vi "Parameters Import Action - Create Chans.v.vi"(8 "error in (no error)":errorcluster, 9 "Param ID map":map{i32, string}(c390), 10 "selected path":path, 11 "Item Ref in":T1 format="%.0x") -> (0 "error out":errorcluster, 2 "selected path out":path caption="selected path", 3 "Item Ref out":T1 format="%.0x")   [LabVIEW 2020, in "Ballard 1553 System Explorer.lvlib"]
uses:
  Ballard 1553 System Explorer.lvlib
  Shared/Controls and Global/Global.vi
  Shared/Ballard 1553 Shared.lvlib
  <vilib>/NI VeriStand/Custom Device Tools/Custom Device Utility Library/Custom Device Utility Library.lvlib
  <vilib>/NI VeriStand/Custom Device API/Custom Device API.lvlib
  c73aaead-b91a-4278-bfe3-fb22b68f848a.vi
  <vilib>/NI VeriStand/Custom Device Tools/Custom Device Utility Library/NI VeriStand - Search for All Items by GUID.vi
  1876eacf-d948-401b-a296-273bf559280d.vi
  <vilib>/NI VeriStand/Custom Device API/Custom Device Item Ref.ctl
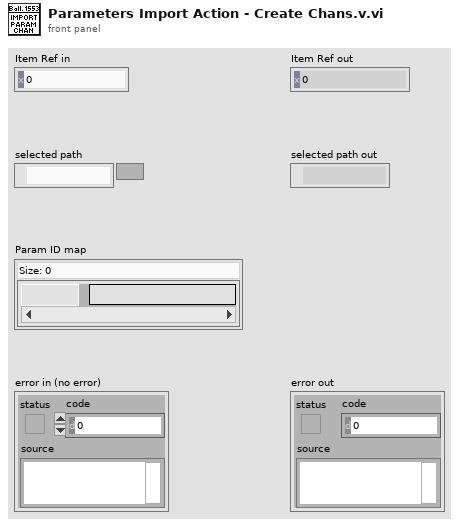
[diagram p1: front panel]
types:
  T1 = typedef "Custom Device API.lvlib/Custom Device Item Ref.ctl" = u64
  T2 = typedef "Ballard 1553 System Explorer.lvlib/param_sysdef_type.ctl" = cluster{"Num_Words":u8, "IDs":string[], "Parameter Map":map{string, cluster{"ICD_Signal_Name":string, "Type":enum16{"Opaque", "Enum", "Float", "Integer", "Bcd", "Bool"}, "Units":string, "Nword":i32, "StartBit":i32, "Size":i32, "LSB_Value":dbl, "Offset":i32, "Encoding":enum16{"None", "2-complement", "Unsigned"}}[]}}
  T3 = typedef "Custom Device API.lvlib/Custom Device Item Info.ctl" = cluster{"Name":string, "Is Channel":bool, "GUID":string, "Is Waveform":bool}
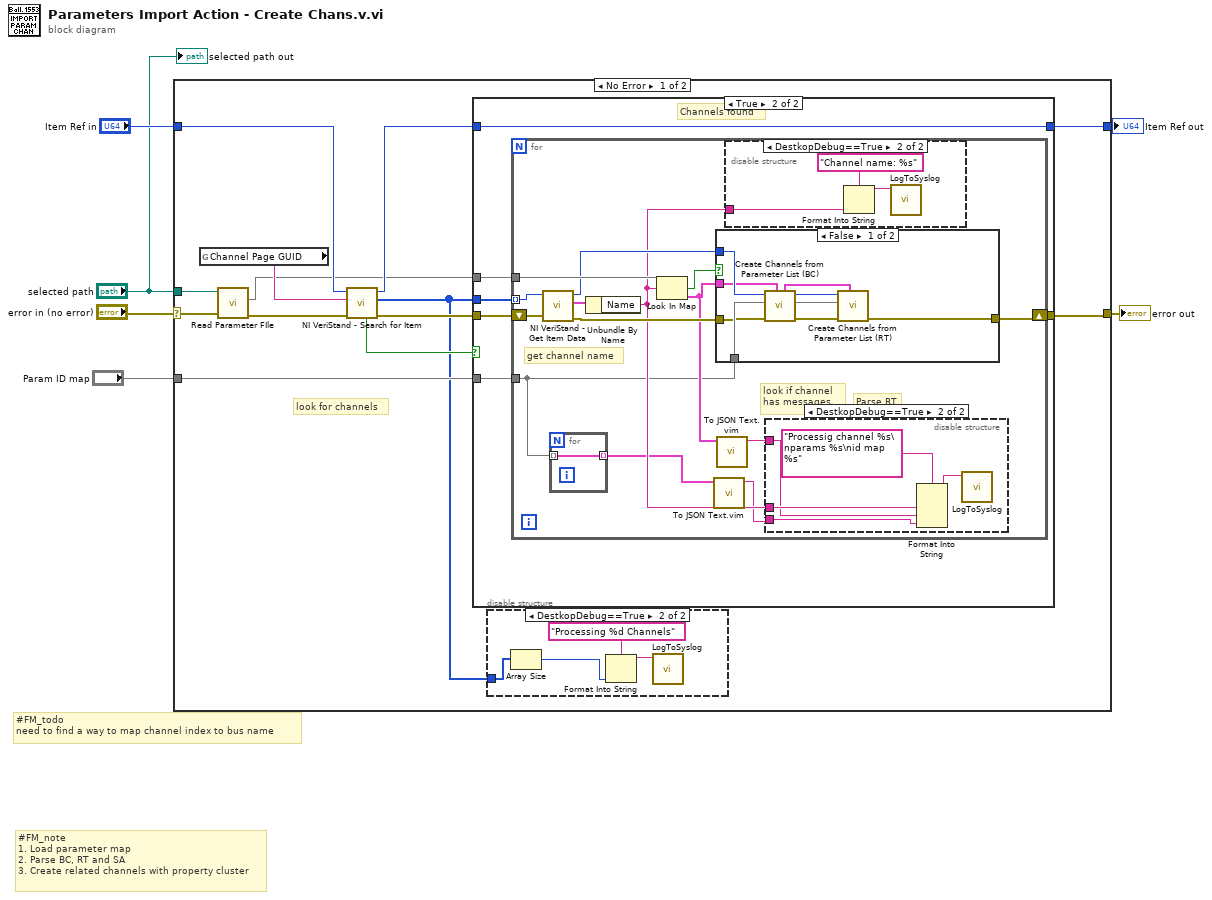
[diagram p0: block diagram]
diagram:
  # "#FM_todo\nneed to find a way to map channel index to bus name"
  # "#FM_note \n1. Load parameter map\n2. Parse BC, RT and SA\n3. Create related channels with property cluster"
  n1 = case shown="No Error" "error in (no error)" {
    selector: "error in (no error)" -> [w18 w65]
    tunnel: "selected path" -> [w19 _]
    tunnel: [w9 w66] -> w5
    tunnel: "Item Ref in" -> [w17 w66]
    tunnel: [w10 w65] -> w3
    tunnel: "Param ID map" -> [w11 _]
    frame No Error {
      # "look for channels"
      n2 = global read "Global.vi" "Channel Page GUID"() -> (w15:string)
      n3 = call "Read Parameter FIle.vi"("error in"=w18, "path in"=w19) -> ("error out"=w16:errorcluster, "Parameter map"=w8:map{string, T2})  [unwired: 7 in, 1 out]
      n4 = call-poly <vilib>:"NI VeriStand - Search for Item.vi"("error in"=w16, "Item GUID"=w15, "Section Ref in"=w17) -> ("error out"=w12:errorcluster, "Item Refs"=w7:T1[], "Section Ref out"=w14:T1, "Found"=w13:bool)  [unwired: 5 in]
      n5 = case shown="True" w13 {
        tunnel: w14 -> [w24 w27]
        tunnel: w7 -> [_ w30]
        tunnel: w12 -> [w25 w31]
        tunnel: w11 -> [_ w29]
        tunnel: [w25 w28] -> w10
        tunnel: [w24 w27] -> w9
        tunnel: w8 -> [_ w26]
        frame False {
        }
        frame True {
          # "Channels found"
          n6 = for {
            shift-right: [w45] -> w28
            shift-left: w31 -> [w43]
            tunnel: w30 -> [w42] mode=indexing
            tunnel: w29 -> [w35]
            tunnel: w26 -> [w44]
            # "look if channel \nhas messages"
            # "Parse RT"
            # "get channel name"
            n7 = call <vilib>:"NI VeriStand - Get Item Data.vi"("error in (no error)"=w43, "Item Ref in"=w42) -> ("error out"=w39:errorcluster, "Item Info"=w41:T3, "Item Ref out"=w40:T1)  [unwired: 7 out]
            n8 = for {
              tunnel: w35 -> [w46] mode=indexing
              tunnel: [w46] -> w34 mode=indexing
            }
            n9 = Unbundle By Name(w41) -> ("Name"=w36:string)
            n10 = Look In Map(map=w44, key=w36) -> (key not found?=w38:bool, value=w37:T2)  [unwired: 1 in]
            n11 = call "To JSON Text.vim"("Anything"=w34) -> ("<JSON>"=w32:string)  [unwired: 9 in, 1 out]
            n12 = case shown="False" w38 {
              tunnel: [w59 w64] -> w45
              tunnel: w35 -> [w63 _]
              tunnel: w40 -> [w62 _]
              tunnel: w39 -> [w61 w64]
              tunnel: w37 -> [w56 _]
              frame False {
                n13 = call "Create Channels from Parameter List (BC).vi"("Message Param map in"=w56, "error in (no error)"=w61, "Param ID map in"=w63, "channel ref in"=w62) -> ("error out"=w60:errorcluster, "Param ID map out"=w57:map{i32, string}, "channel ref out"=w58:T1, "Message Param map out"=w55:T2)  [unwired: 4 in]
                n14 = call "Create Channels from Parameter List (RT).vi"("Message Param map in"=w55, "error in (no error)"=w60, "Param ID map in"=w57, "channel ref in"=w58) -> ("error out"=w59:errorcluster)  [unwired: 4 in, 3 out]
              }
              frame True {
              }
            }
            n15 = call "To JSON Text.vim"("Anything"=w37) -> ("<JSON>"=w33:string)  [unwired: 9 in, 1 out]
            n16 = disable-structure shown="DestkopDebug==True" {
              disable-tunnel: w36 -> [_ w53]
              frame condition #0 {
              }
              frame condition #1 (active) {
                n17 = Format Into String(format string="Channel name: %s", w53) -> (resulting string=w52:string)  [unwired: 2 in, 1 out]
                n18 = call "LogToSyslog.vi"("message"=w52) -> ()  [unwired: 9 in, 2 out]
              }
            }
            n19 = disable-structure shown="DestkopDebug==True" {
              disable-tunnel: w36 -> [_ w49]
              disable-tunnel: w33 -> [_ w48]
              disable-tunnel: w32 -> [_ w47]
              frame condition #0 {
              }
              frame condition #1 (active) {
                n20 = Format Into String(format string="Processig channel %s\nparams %s\nid map %s", w49, w48, w47) -> (resulting string=w50:string)  [unwired: 2 in, 1 out]
                n21 = call "LogToSyslog.vi"("message"=w50) -> ()  [unwired: 9 in, 2 out]
              }
            }
          }
        }
      }
      n22 = disable-structure shown="DestkopDebug==True" {
        disable-tunnel: w7 -> [_ w22]
        frame condition #0 {
        }
        frame condition #1 (active) {
          n23 = Array Size(array=w22) -> (size(s)=w21:i32)
          n24 = Format Into String(format string="Processing %d Channels", w21) -> (resulting string=w20:string)  [unwired: 2 in, 1 out]
          n25 = call "LogToSyslog.vi"("message"=w20) -> ()  [unwired: 9 in, 2 out]
        }
      }
    }
    frame Error {
    }
  }
  "error out" <- w3
  "Item Ref out" <- w5
  "selected path out" <- "selected path"
